vi "IntegratorStage1.vi"(10 "input valid":bool, 11 "data in":bool[](array[boolean])) -> (2 "output valid":bool, 3 "data out":bool[](array[boolean]))   [LabVIEW 2011]
uses:
  <vilib>/rvi/FXPMathLib/basic elements/FxpIntAccumulator/simVIs/DllFxpIntAccumulator_sub.vi
  <vilib>/rvi/FXPMathLib/basic elements/FxpDiscreteDelay/XNode/nifxpmath_DiscreteDelay.xnode
  <vilib>/rvi/FXPMathLib/basic elements/FxpIntAccumulator/XNode/nifxpmath_IntAccumulator.xnode
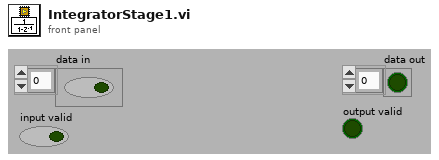
[diagram p1: front panel]
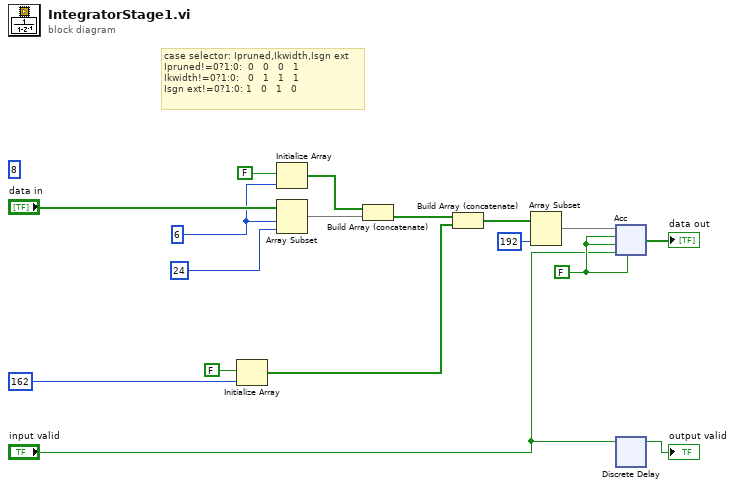
[diagram p0: block diagram]
diagram:
  w2 = 6 ("kIntegratorPruned")
  w15 = FALSE ("load")
  (unwired) 8 ("kCaseSel")
  # "case selector: Ipruned,Ikwidth,Isgn ext\nIpruned!=0?1:0:  0   0   0   1\nIkwidth!=0?1:0:   0   1   1   1\nIsgn ext!=0?1:0: 1   0   1   0"
  n1 = Initialize Array(FALSE, 162 ("kIntegrator192-MaxWidth")) -> (w9:bool[])
  n2 = Initialize Array(FALSE, w2) -> (w3:bool[])
  n3 = Array Subset(array="data in", index=w2, length=24 ("kIntegratorWidth")) -> (w5:bool[])
  n4 = Build Array (concatenate)(w3, w5) -> (w10:bool[])
  n5 = Build Array (concatenate)(w10, w9) -> (w8:bool[])
  n6 = Array Subset(array=w8, length=192) -> (w7:bool[])  [unwired: 1 in]
  n7 = xnode ("Acc")("x"=w7, "load (F)"=w15, "is sub? (F)"=w15, "enable (T)"="input valid", "carry-in/inverted borrow-in (F)"=w15) -> ("s"=→"data out":bool[])  [unwired: 1 out]
  n8 = xnode ("Discrete Delay")("D"="input valid") -> ("Q"=→"output valid":bool)
